vi "Triggers Construct.vi"(6 "triggerable frames":T1[](array[typedef]) {"Acyclic Messages"."Timestamp Channel Handle" format="%.0x"; "Acyclic Messages"."Message Section Handle" format="%.0x"; "Acyclic Messages"."Parameter Channel Handles" format="%.0x"}, 8 "error in":errorcluster, 10 "biu configuration":T6, 11 "id":string) -> (0 "error out":errorcluster, 3 "triggers execution unit":refnum<class "Triggers Execution Unit.lvclass">)   [LabVIEW 2020, in "AIM MIL-STD-1553 Engine.lvlib" / "Implementation.lvlib" / "Triggers Execution Unit.lvclass"]
uses:
  Triggers Execution Unit.lvclass
  Execution Unit/Execution Unit.lvclass
  Shared/Running Status.ctl
  C:/dev/git/niveristand-aim-milStd1553-custom-device/Source/Custom Device Support/Engine/Implementation/Execution Unit/Execution Unit.lvclass
  C:/dev/git/niveristand-aim-milStd1553-custom-device/Source/Custom Device Support/Engine/Interfaces/Execution Unit/Execution Unit.lvclass
  C:/dev/git/niveristand-aim-milStd1553-custom-device/Source/Custom Device Support/Engine/Implementation/Triggers Execution Unit/Triggers Execution Unit.lvclass
  Shared/Address.ctl
  Shared/Terminal Endpoint.ctl
  Shared/Parameter Definition.ctl
  Shared/Message Type.ctl
  Shared/Message Definition.ctl
  Shared/BIU Configuration.ctl
  Shared/Major Frame Definition.ctl
  Shared/Minor Frame Definition.ctl
  Shared/Acyclic Frame Definition.ctl
  Shared/Direction.ctl
  <vilib>/NI VeriStand/Custom Device API/Custom Device Item Ref.ctl
  <vilib>/NI VeriStand/Custom Device API/Custom Device API.lvlib
  Custom Device/Compiled Message.ctl
  Custom Device/Custom Device.lvlib
  Triggerable Frame.ctl
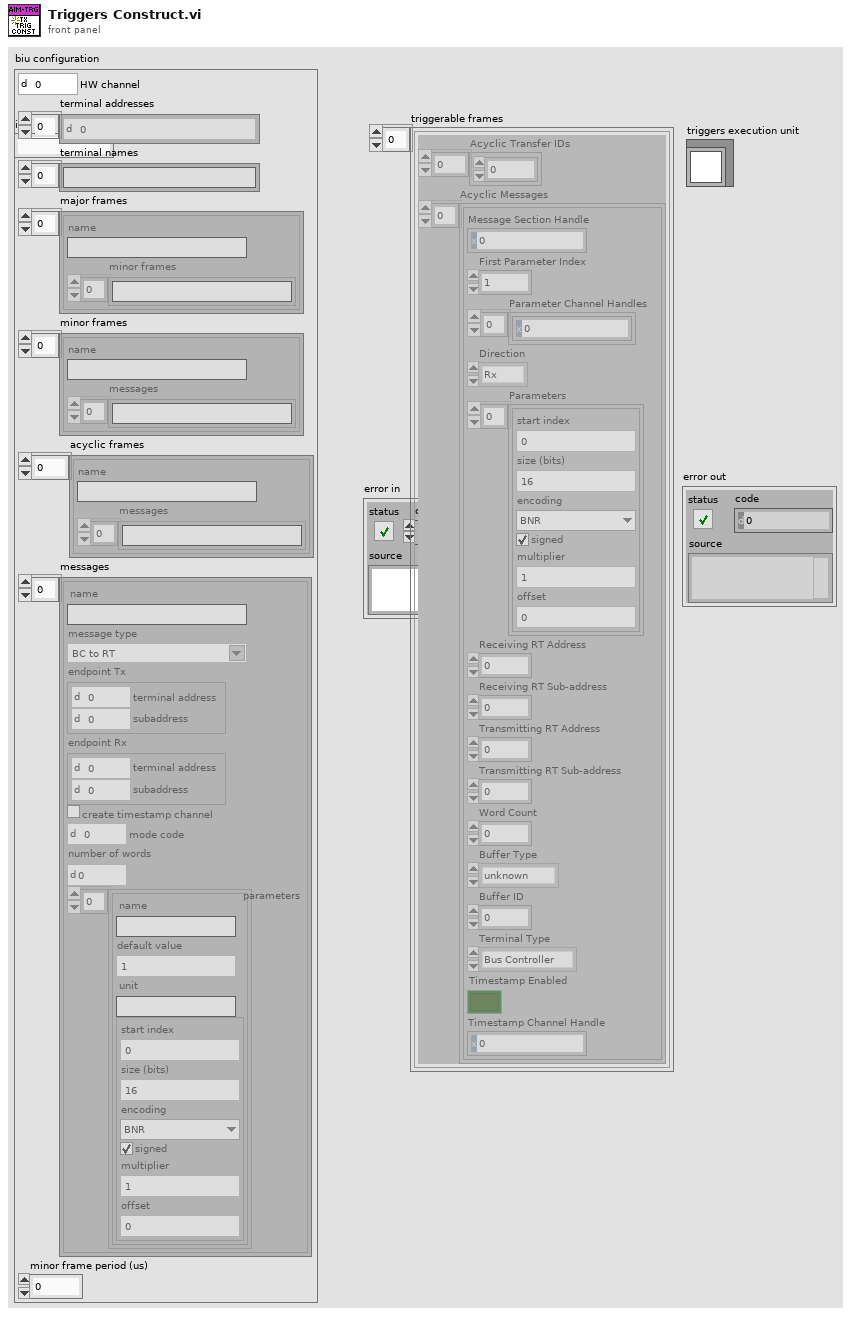
[diagram p1: front panel]
types:
  T1 = typedef "AIM MIL-STD-1553 Engine.lvlib/Implementation.lvlib/Triggers Execution Unit.lvclass/Triggerable Frame.ctl" = cluster{"Acyclic Transfer IDs":u16[], "Acyclic Messages":T2[]}
  T2 = typedef "AIM MIL-STD-1553 Engine.lvlib/Custom Device.lvlib/Compiled Message.ctl" = cluster{"Message Section Handle":T3, "First Parameter Index":i32, "Parameter Channel Handles":T3[], "Direction":T4, "Parameters":T5[], "Receiving RT Address":u8, "Receiving RT Sub-address":u8, "Transmitting RT Address":u8, "Transmitting RT Sub-address":u8, "Word Count":u8, "Buffer Type":enum16{"unknown", "BC Message Buffer", "RT Message Buffer"}, "Buffer ID":u16, "Terminal Type":enum16{"Bus Controller", "Remote Terminal"}, "Timestamp Enabled":bool, "Timestamp Channel Handle":T3}
  T3 = typedef "Custom Device API.lvlib/Custom Device Item Ref.ctl" = u64
  T4 = typedef "Direction.ctl" = enum16{"Rx", "Tx"}
  T5 = typedef "Parameter Definition.ctl" = cluster{"start index":i32, "size (bits)":i32, "encoding":enum16{"BNR", "BCD", "Discrete"}, "signed":bool, "multiplier":dbl, "offset":dbl}
  T6 = typedef "BIU Configuration.ctl" = cluster{"HW channel":u16, "terminal addresses":T7[], "terminal names":string[], "major frames":T8[], "minor frames":T9[], "acyclic frames":T10[], "messages":T11[], "minor frame period (us)":i32}
  T7 = typedef "Address.ctl" = u16
  T8 = typedef "Major Frame Definition.ctl" = cluster{"name":string, "minor frames":string[]}
  T9 = typedef "Minor Frame Definition.ctl" = cluster{"name":string, "messages":string[]}
  T10 = typedef "Acyclic Frame Definition.ctl" = cluster{"name":string, "messages":string[]}
  T11 = typedef "Message Definition.ctl" = cluster{"name":string, "message type":T12, "endpoint Tx":T13, "endpoint Rx":T13, "create timestamp channel":bool, "mode code":u16, "number of words":u16, "parameters":cluster{"name":string, "default value":dbl, "unit":string, "parameter definition":T5}[]}
  T12 = typedef "Message Type.ctl" = string
  T13 = typedef "Terminal Endpoint.ctl" = cluster{"terminal address":T7, "subaddress":T7}
  T14 = typedef "Running Status.ctl" = enum16{"Running", "Stopped"}
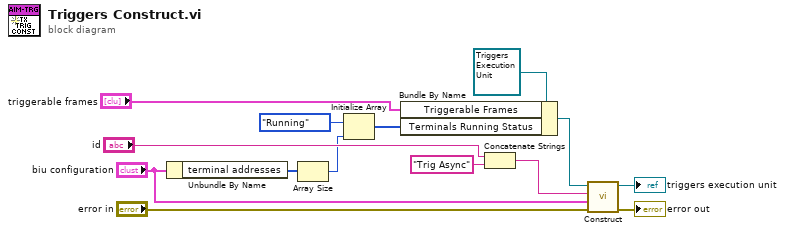
[diagram p0: block diagram]
diagram:
  n1 = Unbundle By Name("biu configuration") -> ("terminal addresses"=w1:T7[])
  n2 = Array Size(array=w1) -> (size(s)=w7:i32)
  n3 = Initialize Array(Running_Status."Running" ("Running Status"), w7) -> (w5:T14[])
  n4 = Bundle By Name(cluster=refnum<class "Triggers Execution Unit.lvclass"> refnum ("Communication Bus Template Interfaces:Implementation.lvlib:Address Based Execution Unit.lvclass"), "Triggerable Frames"="triggerable frames", "Terminals Running Status"=w5) -> (w13:refnum<class "Triggers Execution Unit.lvclass">)
  n5 = Concatenate Strings("id", "Trig Async" ("id")) -> (w10:string)
  n6 = call "Construct.vi"("error in"="error in", "biu configuration"="biu configuration", "id"=w10, "execution unit"=w13) -> ("error out"=→"error out":errorcluster, "execution unit out"=→"triggers execution unit":refnum<class "Triggers Execution Unit.lvclass">)  [unwired: 6 in]
